vi "Tester_VI.vi"(0 "Voltage_Configurations":T1={"Resolution[V]"=0.01, "Maximum[V]"=5.0, "Minimum[V]"=3.0} {"Minimum[V]" step=0.01 format="%#.2g"; "Maximum[V]" step=0.01 format="%#.2g"; "Resolution[V]" min=1e-06 max=1.0 step=0.01}, 11 "Stop":bool) -> (4 "Voltage_Failure_Point(V)":dbl format="%#.8g")   [LabVIEW 2021]
doc: "This VI Rolls over the Voltage range and determine the Fault point at which the Module fails."
uses:
  Controls/Voltage_Configurations.ctl
panel:
  # "FAULT POINT TESTER"
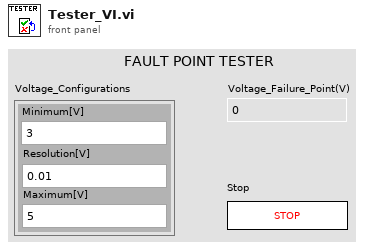
[diagram p1: front panel]
types:
  T1 = typedef "Voltage_Configurations.ctl" = cluster{"Resolution[V]":dbl, "Maximum[V]":dbl, "Minimum[V]":dbl}
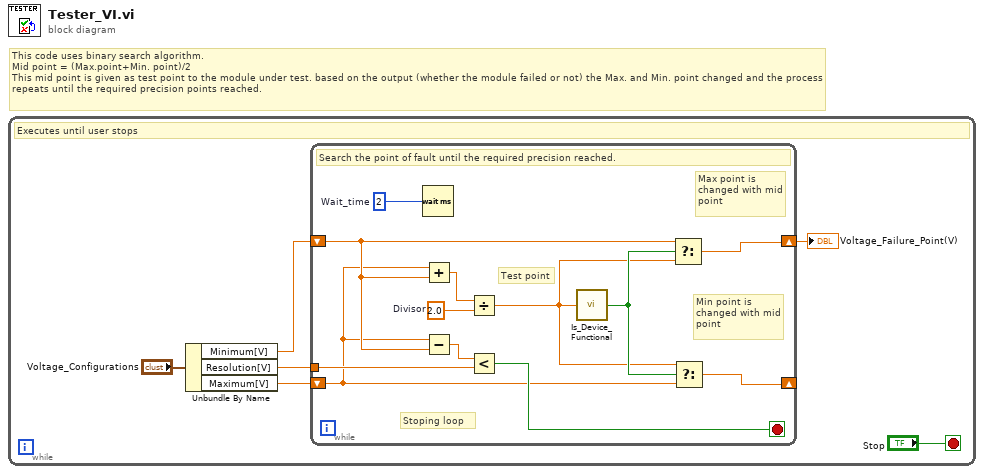
[diagram p0: block diagram]
diagram:
  # "This code uses binary search algorithm.\nMid point = (Max.point+Min. point)/2\nThis mid point is given as test point to the module under test. based on the output (whether the module failed or not) the Max. and Min. point changed and the process repeats until the required precision points reached."
  n1 = while {
    stop <- "Stop" stop-if-true
    # "Executes until user stops"
    n2 = Unbundle By Name("Voltage_Configurations") -> ("Minimum[V]"=w3:dbl, "Resolution[V]"=w2:dbl, "Maximum[V]"=w1:dbl)
    n3 = while {
      shift-right: [w10] -> w6
      shift-left: w3 -> [w11]
      shift-right: [w7] -> _
      shift-left: w1 -> [w8]
      tunnel: w2 -> [w14]
      stop <- w16 stop-if-true
      w13 = u32 2  # Wait_time
      w17 = 2.0  # Divisor
      # "Test point"
      # "Min point is changed with mid point"
      # "Max point is changed with mid point"
      # "Stoping loop"
      # "Search the point of fault until the required precision reached."
      n4 = Wait (ms)(milliseconds to wait=w13) -> ()  [unwired: 1 out]
      n5 = Add(x=w8, y=w11) -> (x+y=w18:dbl)
      n6 = Subtract(x=w8, y=w11) -> (x-y=w15:dbl)
      n7 = Divide(x=w18, y=w17) -> (x/y=w9:dbl)
      n8 = Less?(x=w15, y=w14) -> (x < y?=w16:bool)
      n9 = call "Is_Device_Functional.vi"("Operating_Voltage(V)"=w9) -> ("Device_Functional"=w12:bool)  [unwired: 14 in]
      n10 = Select(t=w11, s=w12, f=w9) -> (s? t:f=w10:dbl)
      n11 = Select(t=w9, s=w12, f=w8) -> (s? t:f=w7:dbl)
    }
    "Voltage_Failure_Point(V)" <- w6
  }
